vi "Strings und Zeitstempel verknuepfen.vi"(8 "String 2 hinzufügen":string, 9 "String 1 hinzufügen":string, 11 "Eingagns String":string) -> (2 "Verknüpfter String":string)   [LabVIEW 2020, in "Auto Kalibrieren.lvlib"]
uses:
  Auto Kalibrieren.lvlib
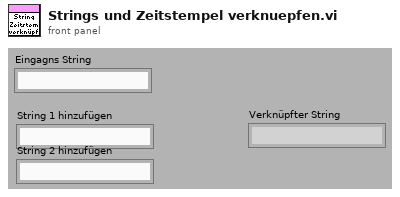
[diagram p1: front panel]
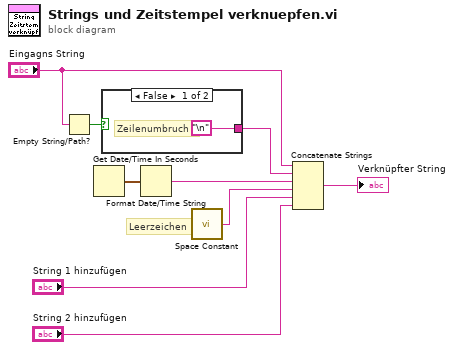
[diagram p0: block diagram]
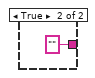
[diagram p2: hidden frame]
diagram:
  # "Leerzeichen"
  n1 = Empty String/Path?(string/path="Eingagns String") -> (empty?=w2:bool)
  n2 = Get Date/Time In Seconds() -> (seconds since 1Jan1904=w8:timestamp)
  n3 = case shown="False" w2 {
    tunnel: ["\n" ""] -> w9
    frame False {
      # "Zeilenumbruch"
    }
    frame True {
    }
  }
  n4 = Format Date/Time String(seconds (now)=w8) -> (date/time string=w7:string)  [unwired: 2 in]
  n5 = call <vilib>:"Space Constant.vi"() -> ("String"=w6:string)
  n6 = Concatenate Strings("Eingagns String", w9, w7, w6, "String 1 hinzufügen", "String 2 hinzufügen") -> (→"Verknüpfter String":string)
